vi "Phase Diff Setup.vi"(7 "Perform Auto Setup":bool, 8 "error in (no error)":errorcluster, 11 "VISA resource name":refnum<visa-resource-name>) -> (0 "error out":errorcluster, 3 "VISA resource name out":refnum<visa-resource-name>)   [LabVIEW 2021]
uses:
  Program Files/National Instruments/LabVIEW 2021/instr.lib/Siglent SDS 1000 2000 Series/Siglent SDS 1000 2000 Series.lvlib
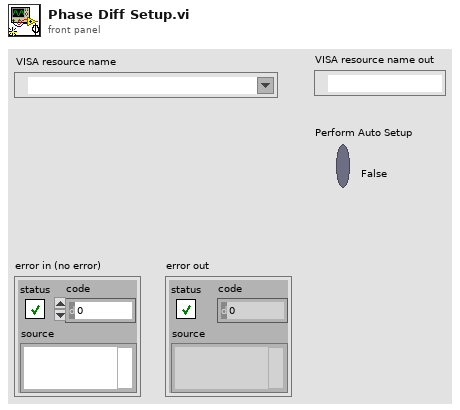
[diagram p1: front panel]
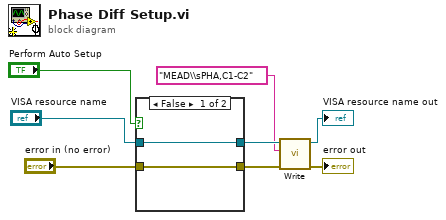
[diagram p0: block diagram]
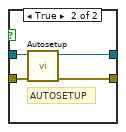
[diagram p2: hidden frame]
diagram:
  n1 = case shown="False" "Perform Auto Setup" {
    tunnel: "error in (no error)" -> [w9 w14]
    tunnel: "VISA resource name" -> [w10 w13]
    tunnel: [w10 w12] -> w5
    tunnel: [w9 w11] -> w4
    frame False {
    }
    frame True {
      # "AUTOSETUP"
      n2 = call "Autosetup.vi"("error in (no error)"=w14, "VISA resource name"=w13) -> ("error out"=w11:errorcluster, "VISA resource name out"=w12:refnum<visa-resource-name>)  [unwired: 8 in]
    }
  }
  n3 = call "Write.vi"("error in (no error)"=w4, "Write Buffer"="MEAD\\sPHA,C1-C2", "VISA resource name"=w5) -> ("error out"=→"error out":errorcluster, "VISA resource name out"=→"VISA resource name out":refnum<visa-resource-name>)  [unwired: 6 in, 1 out]
